vi "GetInfo.vi"(0 "Broker In":u64[](array[numeric]), 2 "DeviceID":u8=1, 6 "error in":errorcluster) -> (12 "error out":errorcluster, 14 "Broker Out":u64[](array[numeric]), 15 "Error":i32, 16 "LastError":i32, 17 "Status":i32, 18 "Connected":bool, 19 "JobTime":i32)   [LabVIEW 2020, in "SnapMB.lvlib"]
uses:
  SnapMB.lvlib
  windows/snapmb.dll
panel:
  out "DeviceStatus":i32[](array[numeric])
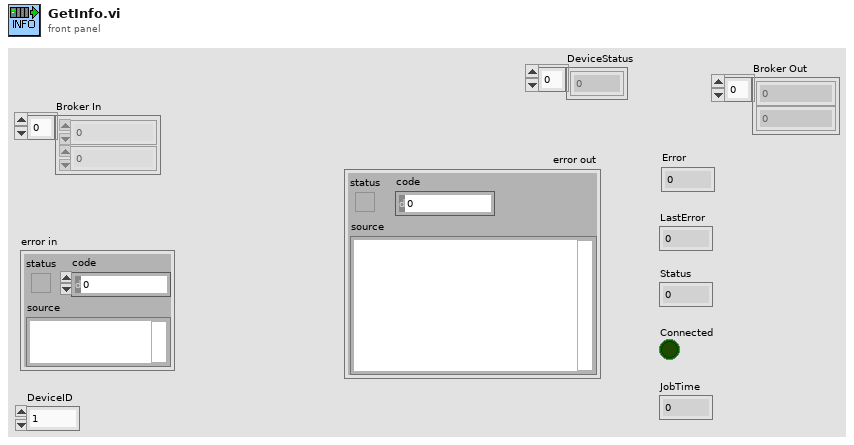
[diagram p1: front panel]
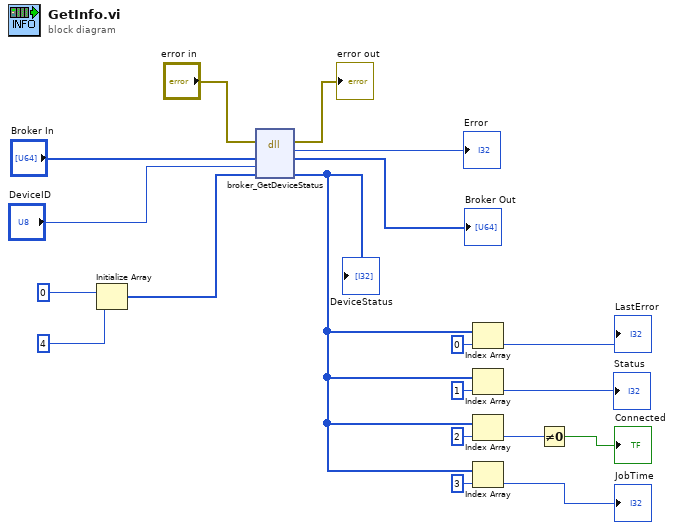
[diagram p0: block diagram]
diagram:
  n1 = Initialize Array(0 ("element"), 4 ("dimension size")) -> (w1:i32[])
  n2 = dll-call lib="D:/SnapMB/LabView/lib/windows/snapmb.dll" fn="broker_GetDeviceStatus"(error in="error in", "Broker"="Broker In", "DeviceID"="DeviceID", "DeviceStatus"=w1) -> (error out=→"error out":errorcluster, "Result"=→"Error":i32, "Broker"=→"Broker Out":u64[], "DeviceStatus"=w9:i32[])  [unwired: 3 in, 1 out]
  "DeviceStatus" <- w9
  n3 = Index Array(array=w9, index=0) -> (element=→"LastError":i32)
  n4 = Index Array(array=w9, index=1) -> (element=→"Status":i32)
  n5 = Index Array(array=w9, index=2) -> (element=w4:i32)
  n6 = Index Array(array=w9, index=3) -> (element=→"JobTime":i32)
  n7 = Not Equal To 0?(x=w4) -> (x != 0?=→"Connected":bool)
